vi "DataProcess_CutAndAverage.vi"() -> ()   [LabVIEW 2015]
uses:
  Shared Libraries/CustomVIs/CustomVI.lvlib
  ExpData/ExpData.lvclass
  <vilib>/Utility/miscctls.llb/LVAnnotationListTypeDef.ctl
  EMG/EMG.lvclass
  CAlex2-Data/CAlex2_Data.lvclass
  TypeDef/Control 1.ctl
panel:
  in  "SyncIn":bool
  out "EMGmean":dbl[][](array[numeric])
  in  "Scale(x1)":u16(ring)=15 items=["x1"=1, "x15"=15]
  out "MuscleNum":i32
  in  "FolderOpen":bool
  in  "Tab Control":enum32{"Cut&Average", "Data Process"}(tab)
  in  "EMG Y scale":i32(slide) min=0 max=1000 step=50 scale=0.0..1000.0
  in  "EMGmean-shift":i32(slide) scale=-100.0..100.0
  in  "Reset Display":bool
  in  "Graph-JointAngles":dbl[][](graph)
  out "GaitTraj":cluster{"Mean":dbl[], "Mean":dbl[]}[](graph)
  in  "Graph-EMG":dbl[][](graph)
  in  "SAVE":bool
  in  "Next":bool
  out "EMGmean-display":dbl[][](graph)
  out "AnglesCutted":dbl[][](graph)
  in  "Cur Parameter":dbl=100.0
  in  "Cut Data":bool
  in  "Cut Method":enum16{"Peak", "Valley", "Threshold"}(ring)
  in  "Graph-AnklePos":dbl[][](graph)
  out "Cycle#":dbl format="%#.1f"
  in  "Start Time (s)":dbl=100.0
  in  "End Time (s)":dbl=100.0
  in  "CutVar":enum16{"3D-x", "2D-x"}(ring)
  in  "Open Gait Template":bool
  in  "Gait Template":path
  out "XY Graph":cluster{"X":dbl, "Y":dbl}[](graph)
  in  "EMG":bool
  in  "Save":bool
  out "EMGstd":dbl[][](array[numeric])
  in  "Overwrite":bool
  in  "Search Pattern":string="sub*.txt"
  in  "Output Folder: Averaged & EMG Files":path=path "E:/Dropbox (Lab)/C-ALEX/Experiments"
  in  "Output Folder: Marked Files":path=path "E:/Dropbox (Lab)/C-ALEX/Experiments"
  in  "File List":i32(listbox)
  in  "FolderStop":bool
  in  "EMG":path
  in  "Unmarked Files":path
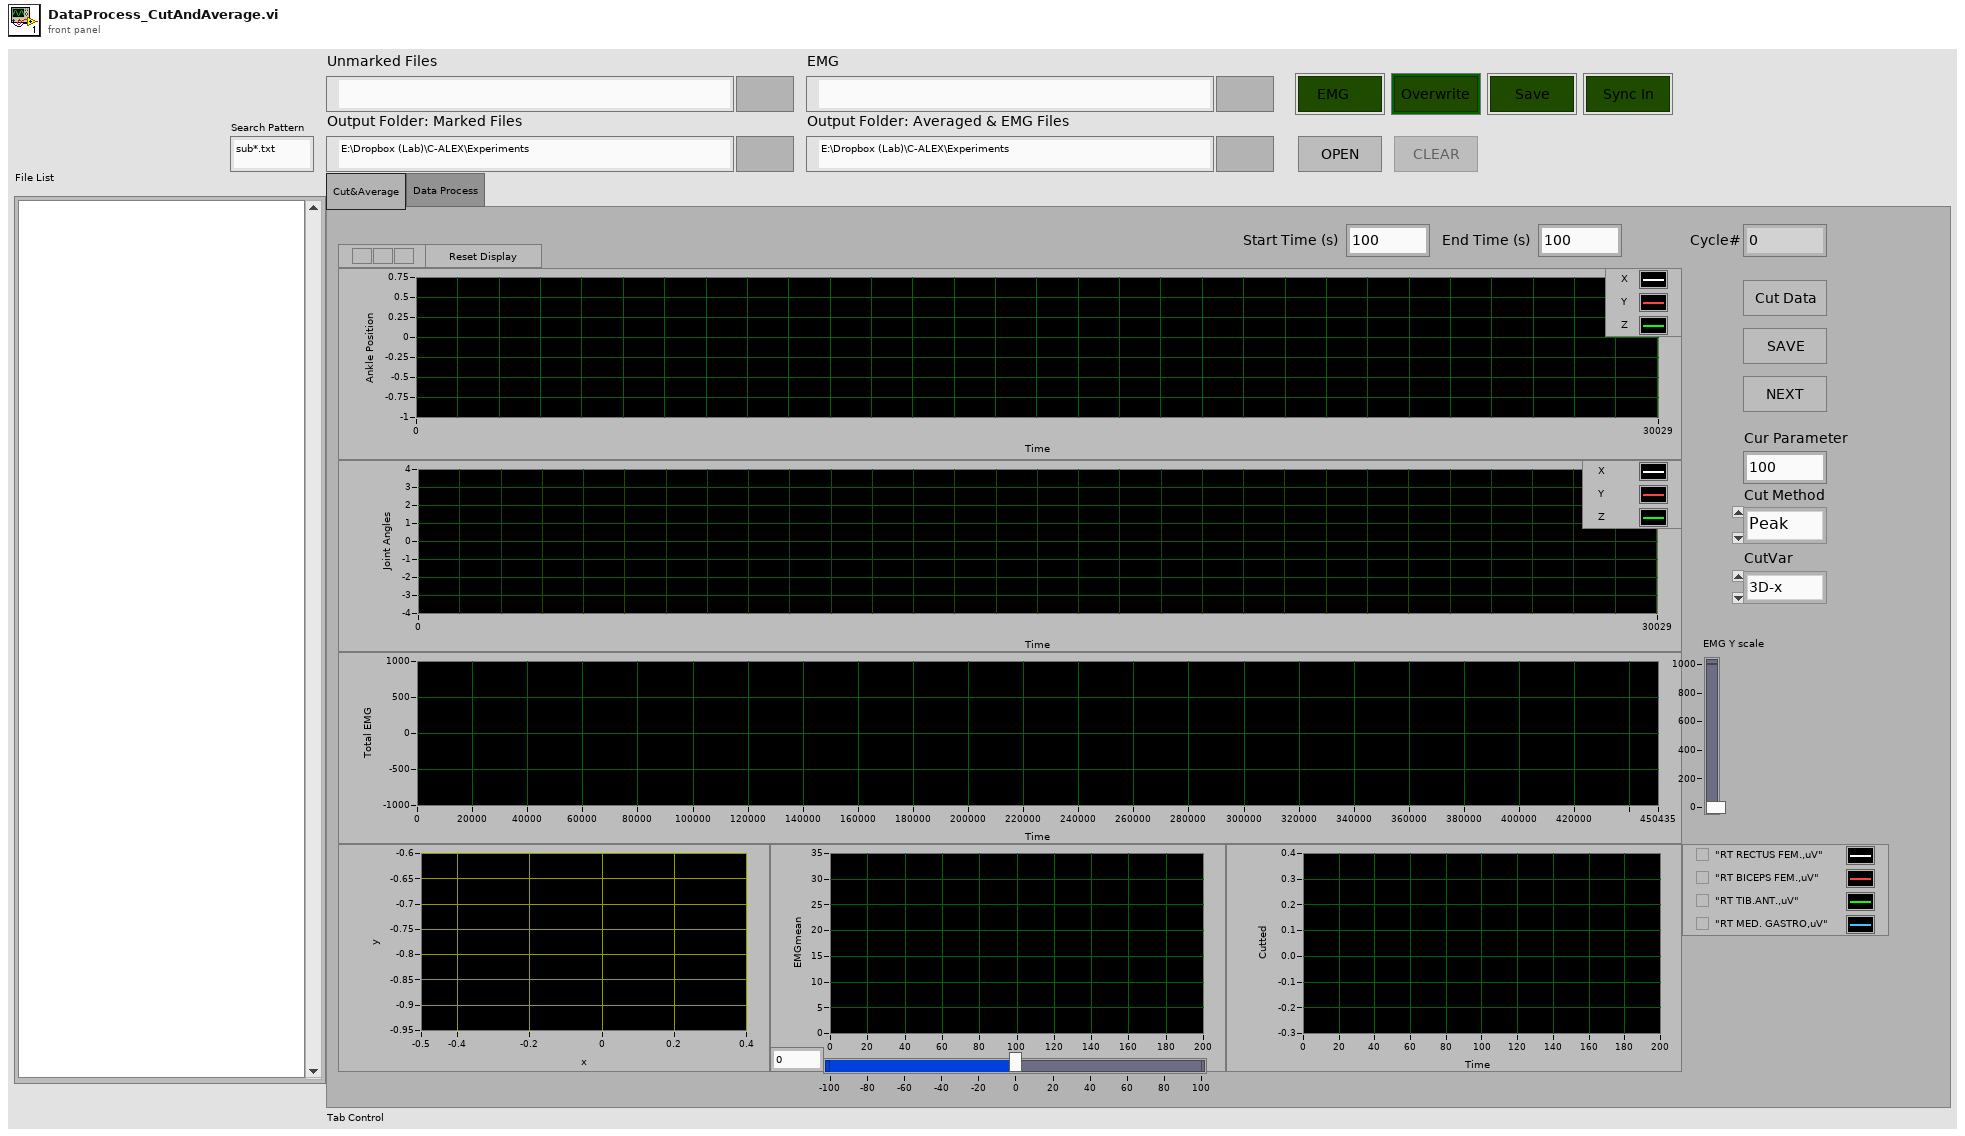
[diagram p1: front panel]
types:
  T1 = typedef "Control 1.ctl" = cluster{"FilePath":path, "ProcParentPath":path, "ResParentPath":path, "EMGPath":path, "CuttedEMGPath":path, "Cutted":bool, "Processed":bool}
  T2 = enum8{"Enabled", "Disabled", "Disabled and Grayed Out"}
  T3 = typedef "LVAnnotationListTypeDef.ctl" = cluster{"Name":string, "Color":u32, "Style":u8, "Point Style":u8, "Name Visible":bool, "Allow Drag":bool, "Annotation Mode":u32, "Plot":i32, "Index":i32, "Position":cluster{"X":dbl, "Y":dbl}, "X Scale":u32, "Y Scale":u32, "Show Arrow":bool, "Lock Name":bool, "Plot Area":i32, "Label Offset":cluster{"X":dbl, "Y":dbl}}[]
  T4 = typedef "LVPoint32TypeDef.ctl" = cluster{"Horizontal":i32, "Vertical":i32}
  T5 = typedef "eventsource.ctl" = u32
  T6 = typedef "LVRangeTypeDef.ctl" = cluster{"Minimum":dbl, "Maximum":dbl, "Increment":dbl, "Minor Increment":dbl, "Start":dbl}
  T7 = cluster{"CuttedData-Concatenated":dbl[], "CuttedData-Concatenated":dbl[]}
  T8 = cluster{"CuttedData-Concatenated":dbl[], "CuttedData-Concatenated":dbl[]}[]
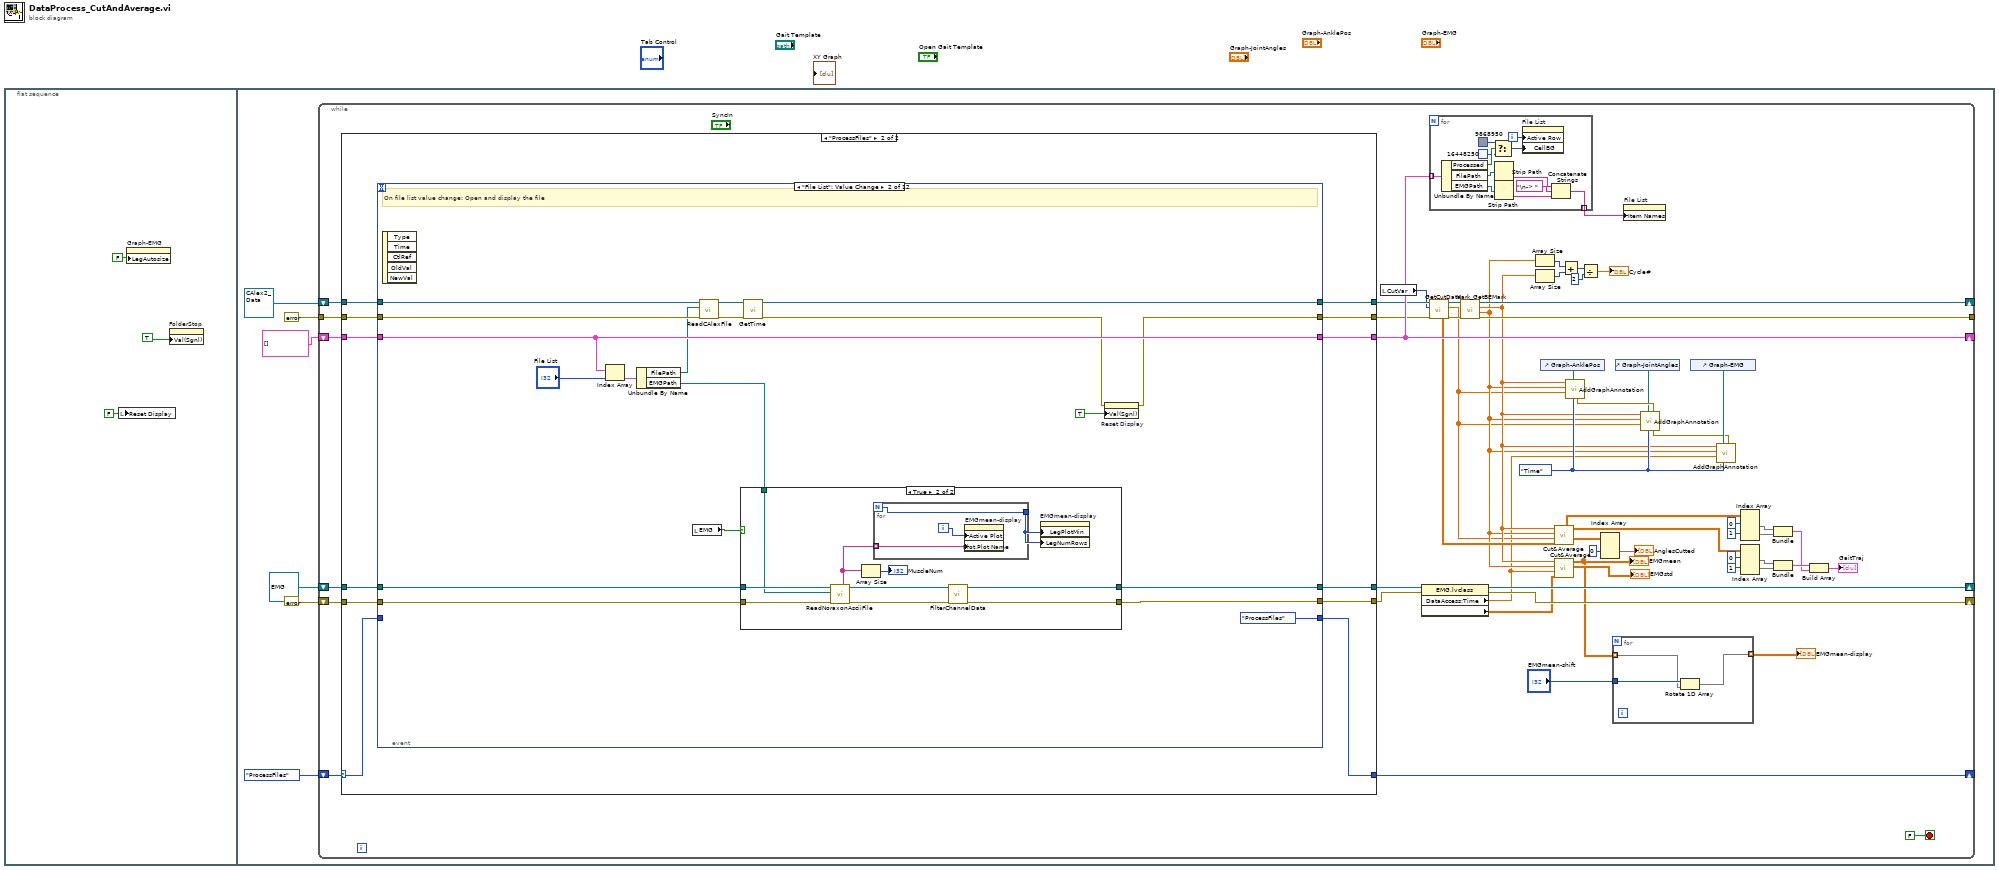
[diagram p0: block diagram]
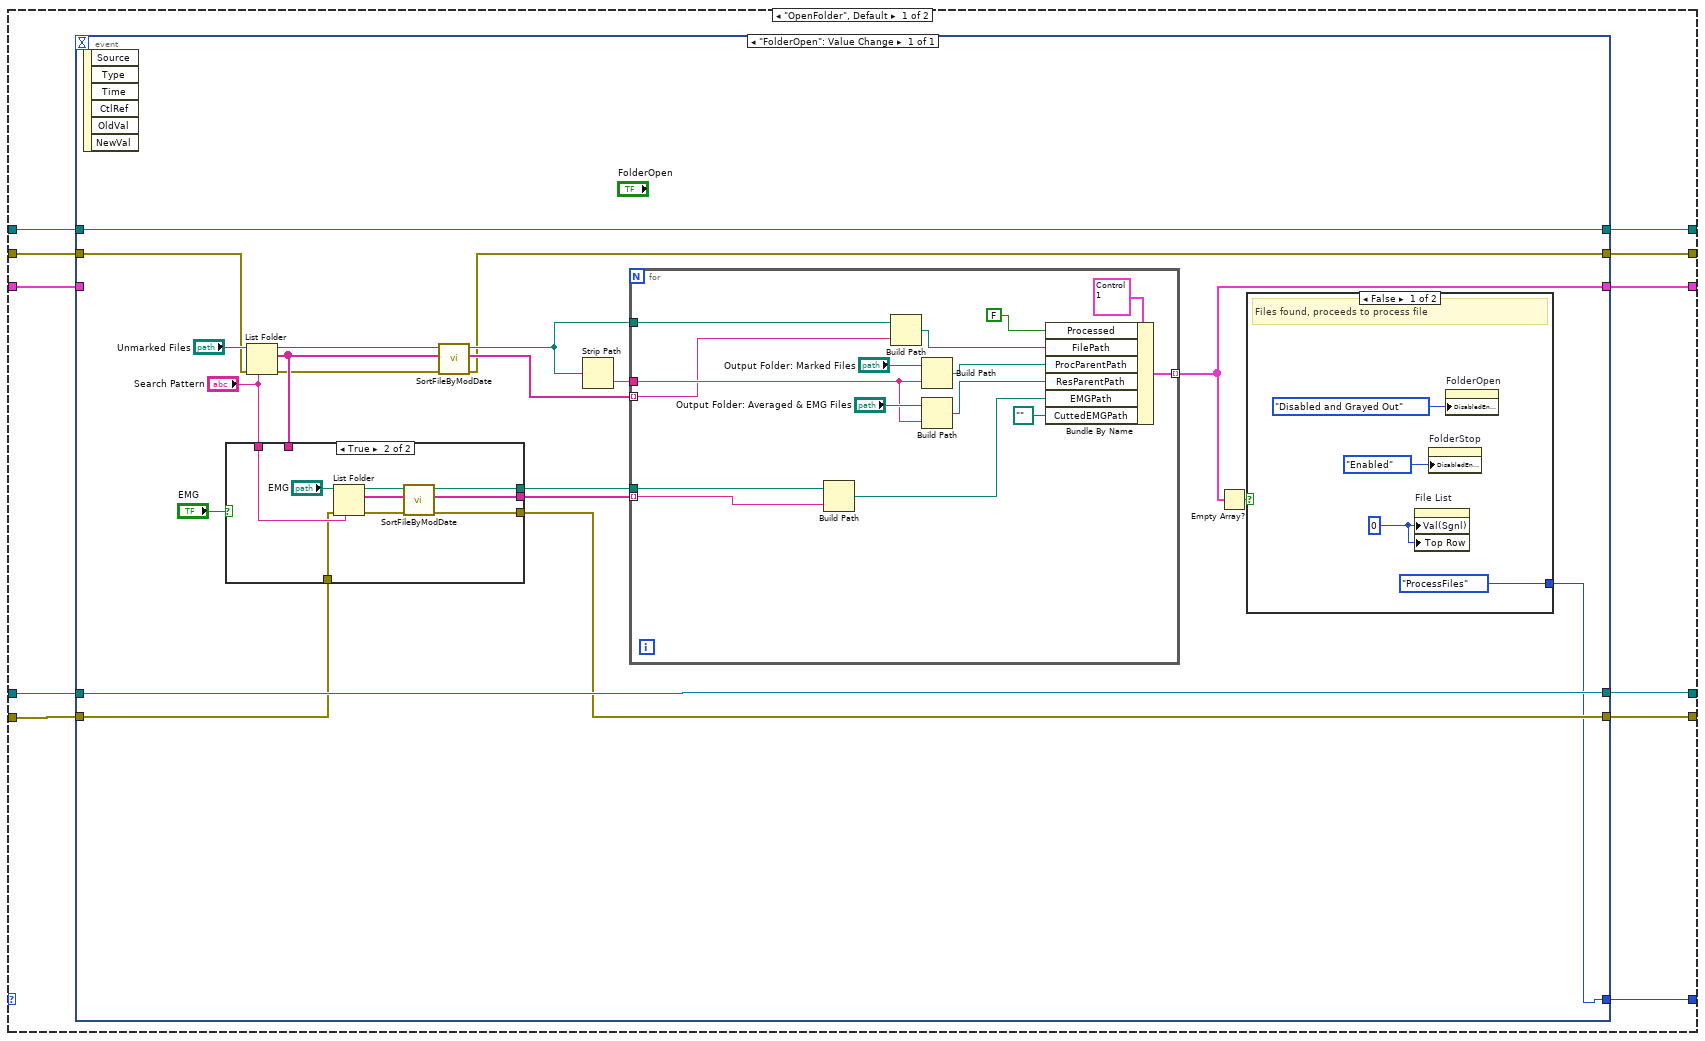
[diagram p2: hidden frame]
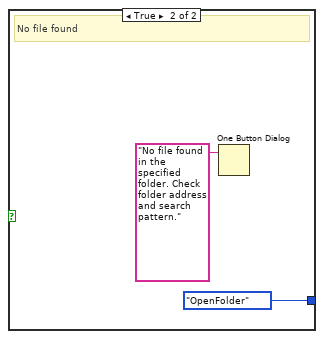
[diagram p3: hidden frame]
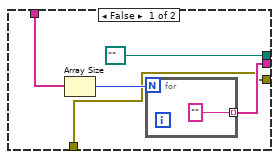
[diagram p4: hidden frame]
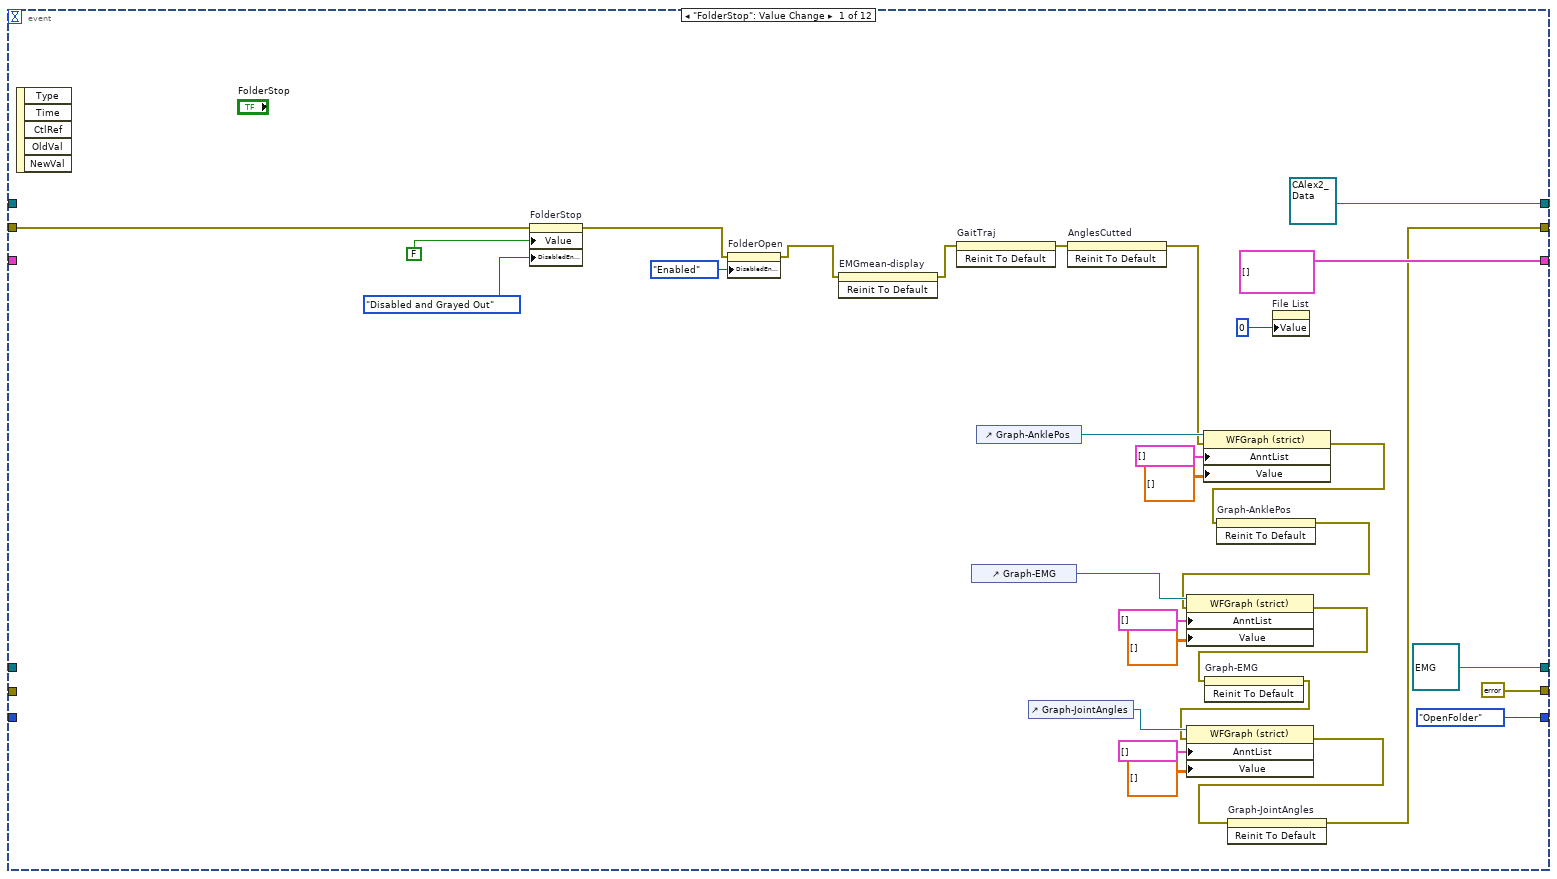
[diagram p5: hidden frame]
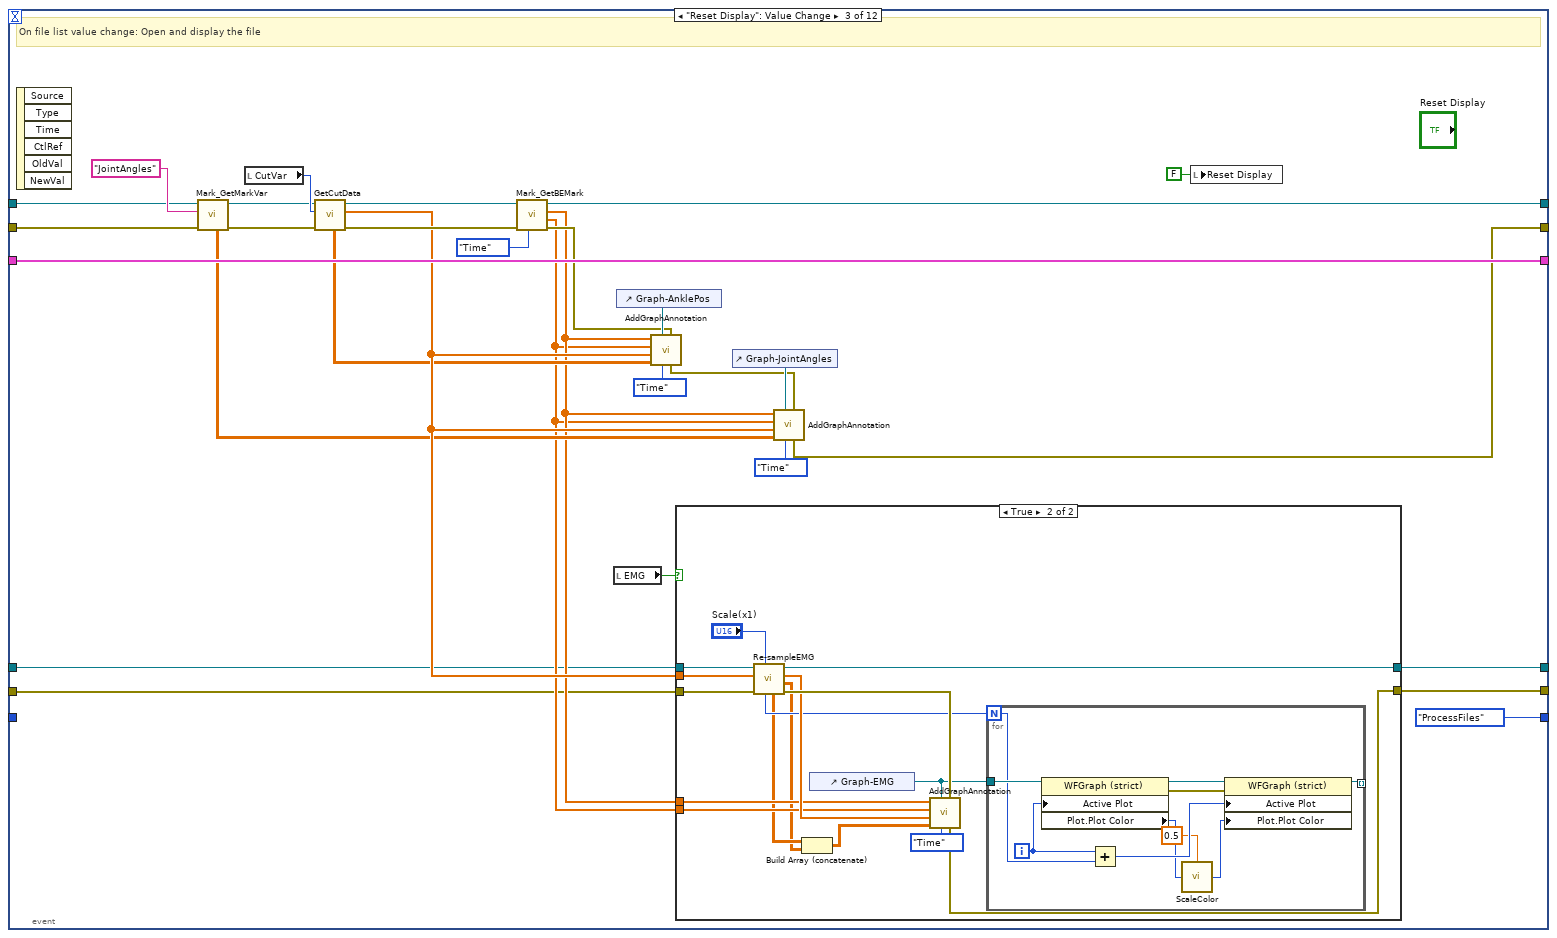
[diagram p7: hidden frame]
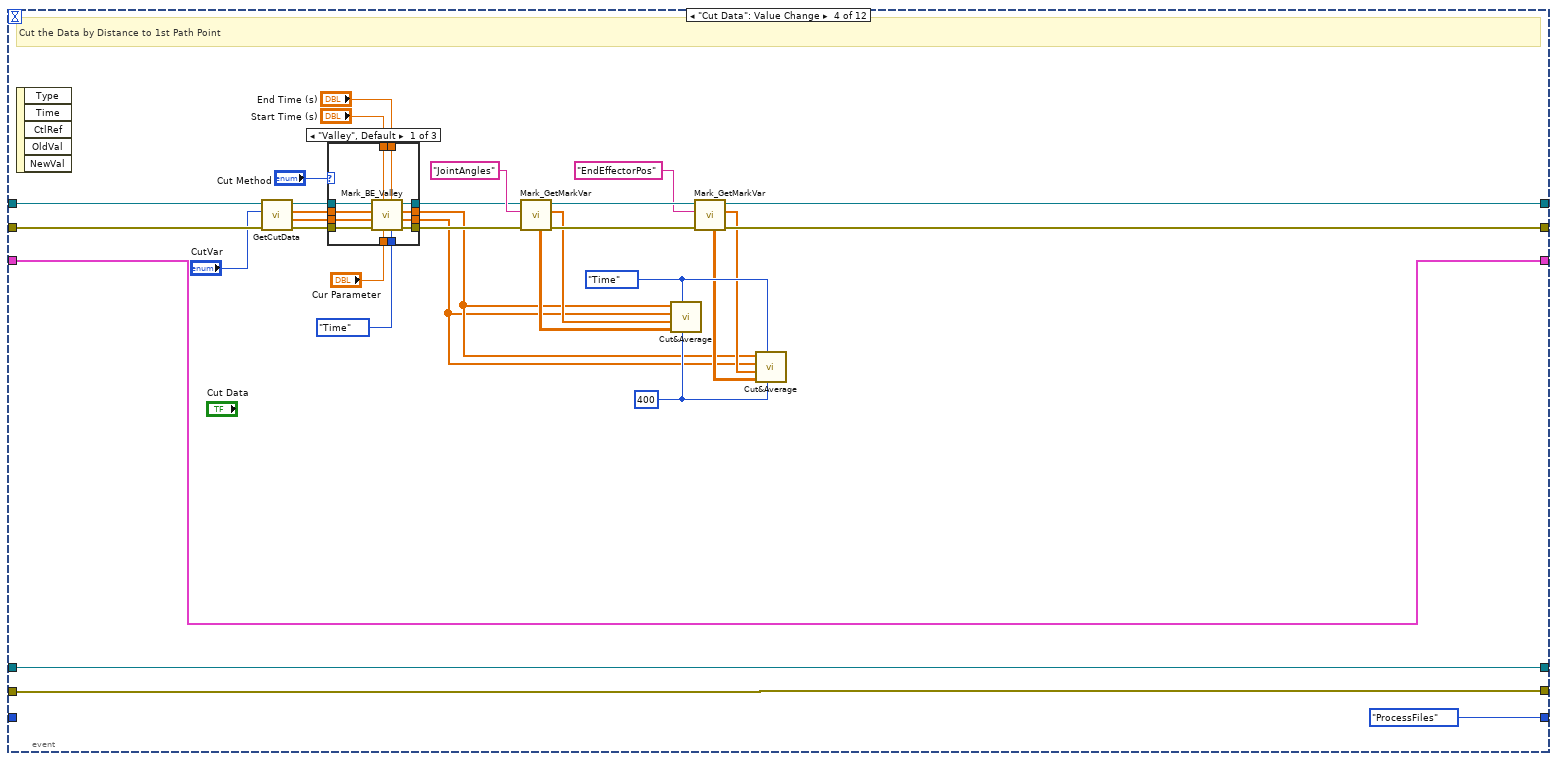
[diagram p9: hidden frame]
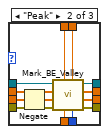
[diagram p10: hidden frame]
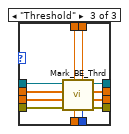
[diagram p11: hidden frame]
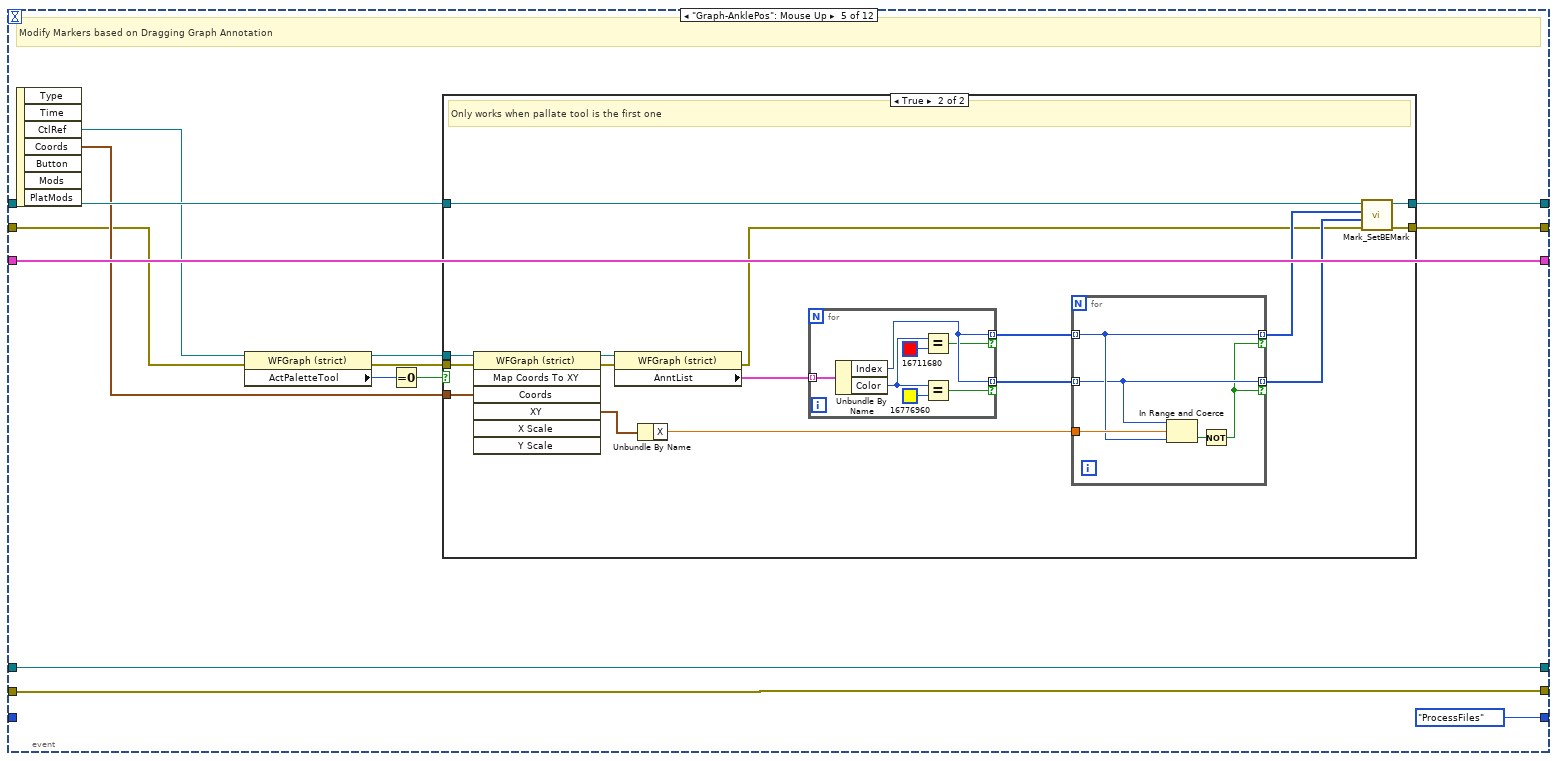
[diagram p12: hidden frame]
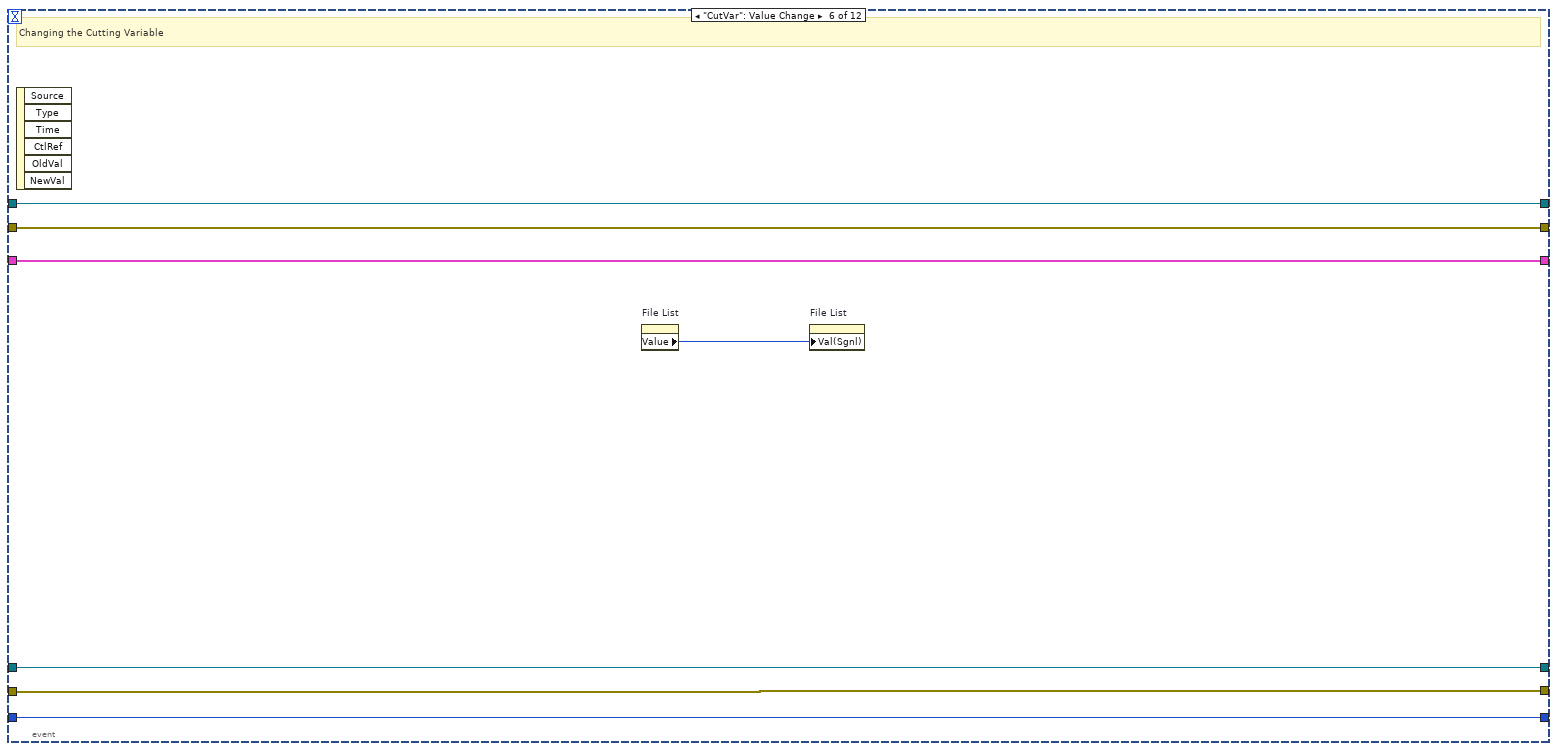
[diagram p14: hidden frame]
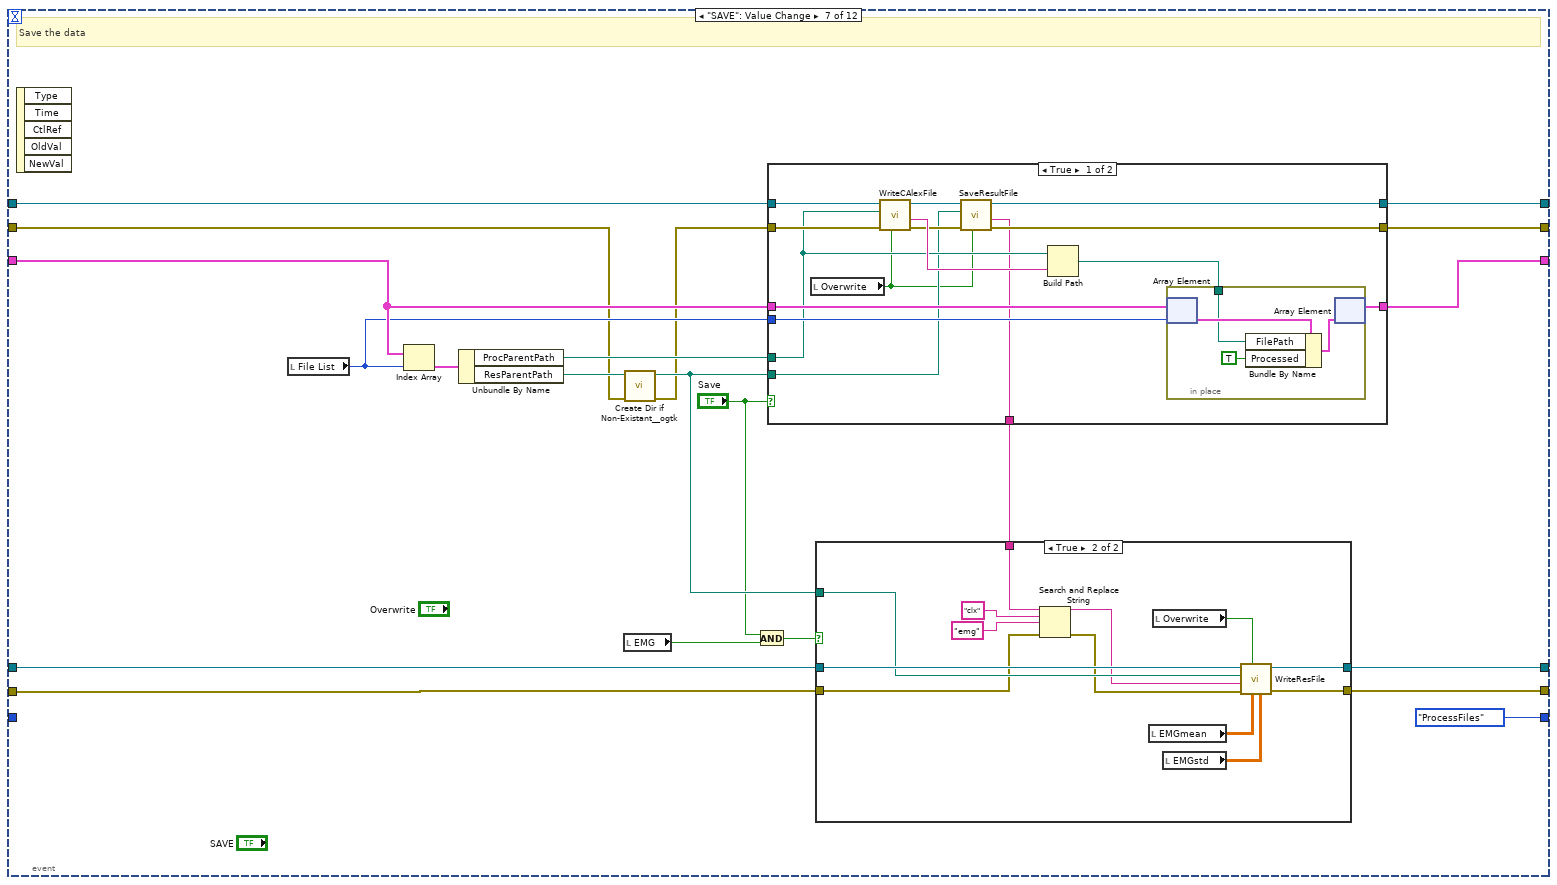
[diagram p15: hidden frame]
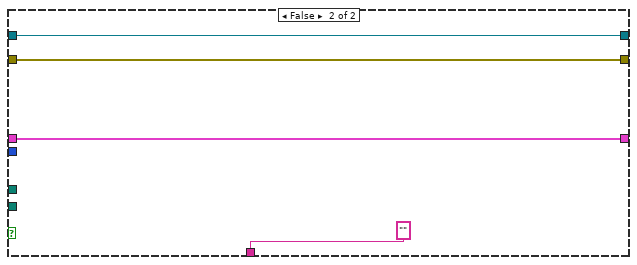
[diagram p17: hidden frame]
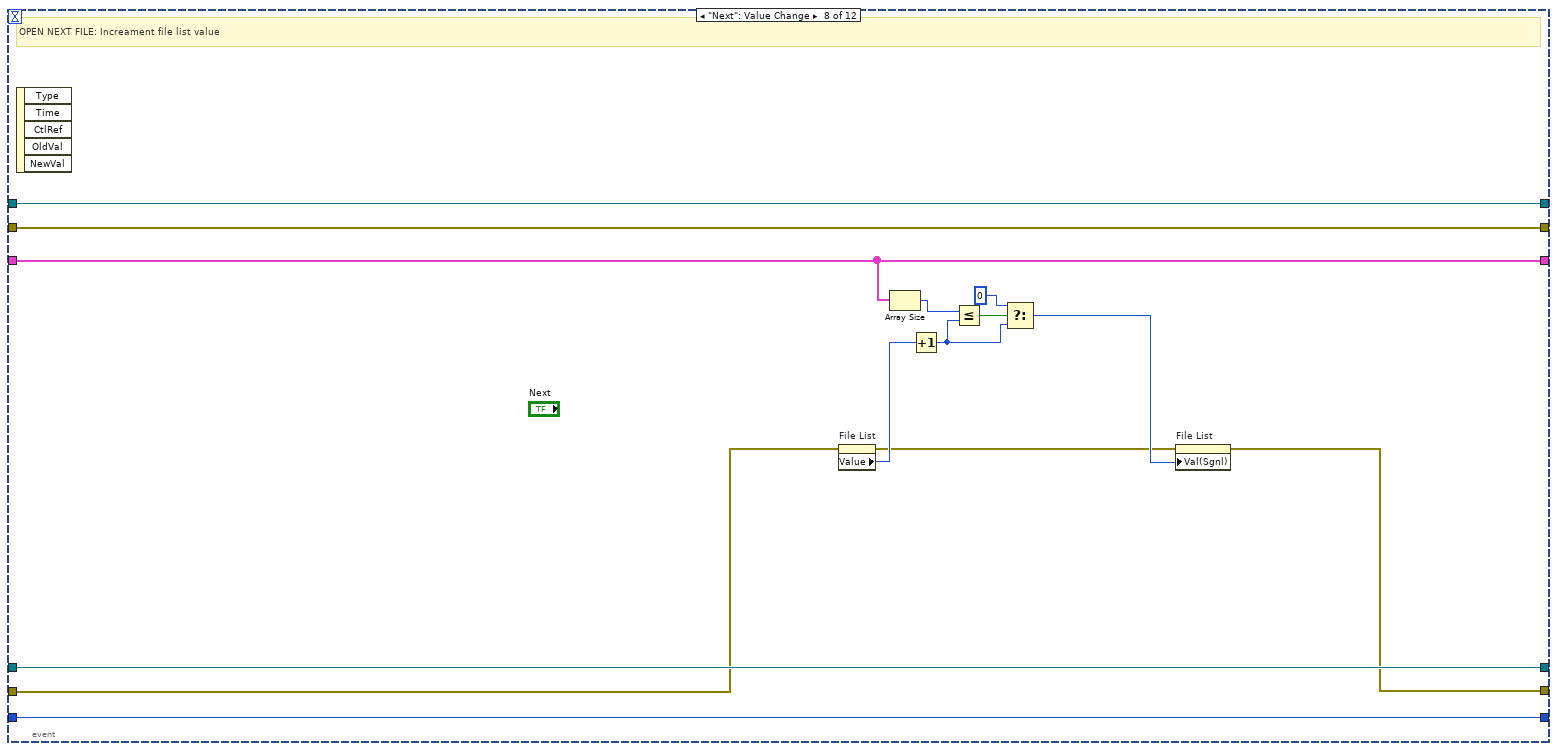
[diagram p18: hidden frame]
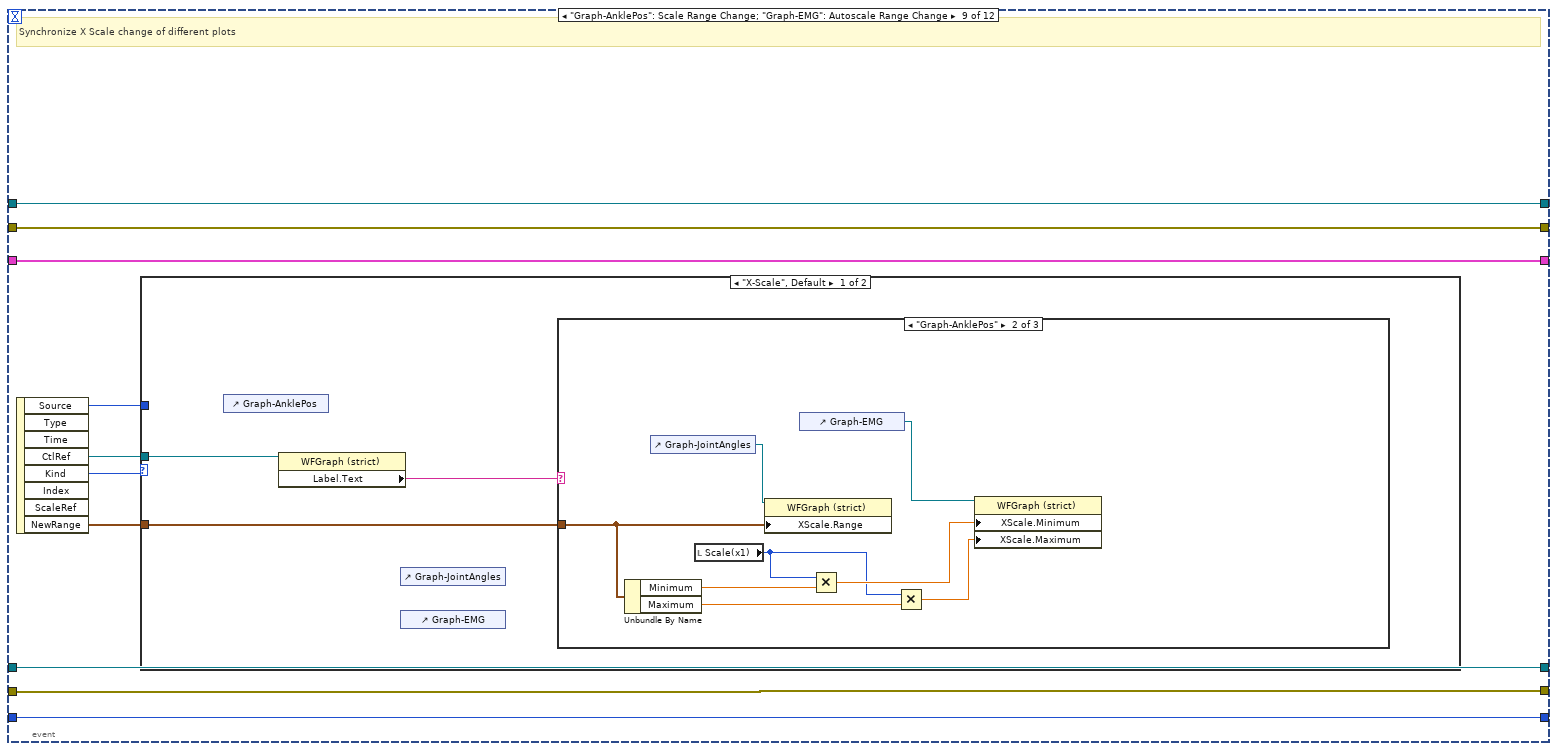
[diagram p19: hidden frame]
diagram:
  n1 = flat-sequence {
    frame #0 {
      n2 = local write "Reset Display"(FALSE ("Reset Display")) -> ()
      n3 = property on="Graph-EMG" class="WFGraph (strict)"("LegAutosize"=FALSE ("Legend:Autosize")) -> ()  [unwired: 2 in, 2 out]
      n4 = property on="FolderStop" class="Bool (strict)"("Val(Sgnl)"=TRUE) -> ()  [unwired: 2 in, 2 out]
    }
    frame #1 {
      n5 = while {
        shift-right: [w61] -> _
        shift-left: enum16{"OpenFolder", "ProcessFiles"}."ProcessFiles" ("State") -> [w39]
        shift-right: [w44] -> _
        shift-left: refnum<class "CAlex2_Data.lvclass"> refnum ("CAlexData") -> [w67]
        shift-right: [w65] -> _
        shift-left: T1[] [] -> [w66]
        tunnel: errorcluster {"status"=FALSE, "code"=0, "source"=""} ("error out") -> [w64]
        tunnel: [w59] -> _
        shift-right: [w54] -> _
        shift-left: refnum<class "EMG.lvclass"> refnum ("EMG.lvclass") -> [w62]
        shift-right: [w52] -> _
        shift-left: errorcluster {"status"=FALSE, "code"=0, "source"=""} ("error out") -> [w60]
        stop <- FALSE stop-if-true
        w18 = enum16{"Time", "Percentage", "Index"}."Time" ("Input Type")
        n6 = case shown="\"ProcessFiles\"" w39 {
          selector: w39 -> [_ w138]
          tunnel: w67 -> [w81 w149]
          tunnel: w66 -> [w79 w148]
          tunnel: [w76 w147] -> w65
          tunnel: w64 -> [w80 w146]
          tunnel: w62 -> [w72 w145]
          tunnel: [w73 w144] -> w61
          tunnel: w60 -> [w71 w143]
          tunnel: [w75 w142] -> w55
          tunnel: [w74 w141] -> w53
          tunnel: [w77 w140] -> w42
          tunnel: [w78 w139] -> w40
          frame "OpenFolder", Default {
            n7 = event shown="[0] \"FolderOpen\": Value Change" {
              selector: _ -> [_]
              dyn-events: _ -> [_]
              timeout: _ -> [_]
              tunnel: w81 -> [w101]
              tunnel: w80 -> [w86]
              tunnel: w79 -> [_]
              tunnel: [w101] -> w78
              tunnel: [w82] -> w77
              tunnel: [w84] -> w76
              tunnel: [w100] -> w75
              tunnel: [w89] -> w74
              tunnel: [w85] -> w73
              tunnel: w72 -> [w100]
              tunnel: w71 -> [w88]
              event "FolderOpen": Value Change {
                n8 = event-data() -> ()  [unwired: 1 in, 6 out]
                n9 = List Folder(path="Unmarked Files", pattern="Search Pattern", error in=w86) -> (path out=w97:path, filenames=w90:string[], error out=w87:errorcluster)  [unwired: 1 in, 1 out]
                n10 = case shown="True" "EMG" {
                  tunnel: [w110 w118] -> w91
                  tunnel: [path "" ("path out") w119] -> w92
                  tunnel: "Search Pattern" -> [_ w121]
                  tunnel: w90 -> [w111 _]
                  tunnel: [w108 w115] -> w89
                  tunnel: w88 -> [w108 w114]
                  frame False {
                    n11 = Array Size(array=w111) -> (size(s)=w109:i32)
                    n12 = for {
                      N: w109 -> [_]
                      tunnel: [""] -> w110 mode=indexing
                    }
                  }
                  frame True {
                    n13 = List Folder(path="EMG", pattern=w121, error in=w114) -> (path out=w120:path, filenames=w117:string[], error out=w116:errorcluster)  [unwired: 1 in, 1 out]
                    n14 = call "SortFileByModDate.vi"("error in (no error)"=w116, "Filenames"=w117, "Parent Path"=w120) -> ("error out"=w115:errorcluster, "Sorted Filenames"=w118:string[], "Parent Path dup"=w119:path)  [unwired: 6 in]
                  }
                }
                n15 = call "SortFileByModDate.vi"("error in (no error)"=w87, "Filenames"=w90, "Parent Path"=w97) -> ("error out"=w82:errorcluster, "Sorted Filenames"=w96:string[], "Parent Path dup"=w95:path)  [unwired: 6 in]
                n16 = Strip Path(path=w95) -> (name=w94:string)  [unwired: 1 out]
                n17 = for {
                  tunnel: w96 -> [w127] mode=indexing
                  tunnel: w91 -> [w123] mode=indexing
                  tunnel: w92 -> [w125]
                  tunnel: w95 -> [w126]
                  tunnel: [w137] -> w84 mode=indexing
                  tunnel: w94 -> [w131]
                  n18 = Build Path(base path=w125, name or relative path=w123) -> (appended path=w124:path)
                  n19 = Build Path(base path=w126, name or relative path=w127) -> (appended path=w128:path)
                  n20 = Build Path(base path="Output Folder: Marked Files", name or relative path=w131) -> (appended path=w134:path)
                  n21 = Build Path(base path="Output Folder: Averaged & EMG Files", name or relative path=w131) -> (appended path=w133:path)
                  n22 = Bundle By Name(cluster=T1 {"FilePath"=path "", "ProcParentPath"=path "", "ResParentPath"=path "", "EMGPath"=path "", "CuttedEMGPath"=path "", "Cutted"=TRUE, "Processed"=FALSE}, "Processed"=FALSE, "FilePath"=w128, "ProcParentPath"=w134, "ResParentPath"=w133, "EMGPath"=w124, "CuttedEMGPath"=path "") -> (w137:T1)
                }
                n23 = Empty Array?(array=w84) -> (empty?=w83:bool)
                n24 = case shown="False" w83 {
                  tunnel: [enum16{"OpenFolder", "ProcessFiles"}."ProcessFiles" ("State") enum16{"OpenFolder", "ProcessFiles"}."OpenFolder" ("State")] -> w85
                  frame False {
                    w105 = 0
                    # "Files found, proceeds to process file"
                    n25 = property on="File List" class="LstBox (strict)"("Val(Sgnl)"=w105, "Top Row"=w105) -> ()  [unwired: 2 in, 2 out]
                    n26 = property on="FolderStop" class="Bool (strict)"("DisabledEnum"=T2."Enabled" ("Disabled")) -> ()  [unwired: 2 in, 2 out]
                    n27 = property on="FolderOpen" class="Bool"("DisabledEnum"=T2."Disabled and Grayed Out" ("Disabled")) -> ()  [unwired: 2 in, 2 out]
                  }
                  frame True {
                    # "No file found"
                    n28 = One Button Dialog(message="No file found in the specified folder. Check folder address and search pattern.") -> ()  [unwired: 1 in, 1 out]
                  }
                }
              }
            }
          }
          frame "ProcessFiles" {
            n29 = event shown="[1] \"File List\": Value Change" {
              selector: _ -> [_ _ _ _ _ _ _ _ _ _ _ _]
              dyn-events: _ -> [_ _ _ _ _ _ _ _ _ _ _ _]
              timeout: _ -> [_ _ _ _ _ _ _ _ _ _ _ _]
              tunnel: [enum16{"OpenFolder", "ProcessFiles"}."OpenFolder" ("State") enum16{"OpenFolder", "ProcessFiles"}."ProcessFiles" ("State") enum16{"OpenFolder", "ProcessFiles"}."ProcessFiles" ("State") enum16{"OpenFolder", "ProcessFiles"}."ProcessFiles" ("State") enum16{"OpenFolder", "ProcessFiles"}."ProcessFiles" ("State") w386 enum16{"OpenFolder", "ProcessFiles"}."ProcessFiles" ("State") w461 w469 w504 w518 w526] -> w144
              tunnel: w149 -> [_ w197 w221 w301 w352 w389 w400 w464 w474 w506 w523 w531]
              tunnel: w148 -> [_ w196 w241 w300 w351 w387 w409 w455 w472 w505 w521 w529]
              tunnel: [T1[] [] w196 w241 w300 w351 w387 w410 w455 w472 w505 w521 w529] -> w147
              tunnel: w138 -> [_ _ _ _ _ w386 _ w461 w469 w504 w518 w526]
              tunnel: [refnum<class "CAlex2_Data.lvclass"> refnum ("CAlexData") w184 w242 w302 w353 w389 w411 w464 w474 w506 w523 w531] -> w139
              tunnel: [w152 w180 w219 w299 w350 w388 w408 w463 w473 w495 w522 w530] -> w140
              tunnel: w146 -> [w161 w195 w220 w298 w344 w388 w394 w463 w473 w496 w522 w530]
              tunnel: w145 -> [_ w194 w215 w297 w349 w390 w406 w462 w471 w501 w520 w528]
              tunnel: w143 -> [_ w193 w214 w296 w348 w391 w404 w452 w470 w499 w519 w527]
              tunnel: [refnum<class "EMG.lvclass"> refnum ("EMG.lvclass") w192 w240 w297 w349 w390 w407 w462 w471 w500 w520 w528] -> w142
              tunnel: [errorcluster {"status"=FALSE, "code"=0, "source"=""} ("error in (no error)") w191 w239 w296 w348 w391 w405 w451 w470 w498 w519 w527] -> w141
              event "FolderStop": Value Change {
                n30 = event-data() -> ()  [unwired: 1 in, 5 out]
                n31 = property on="FolderStop" class="Bool (strict)"(error in=w161, "Value"=FALSE, "DisabledEnum"=T2."Disabled and Grayed Out" ("Disabled")) -> (error out=w160:errorcluster)  [unwired: 1 in, 1 out]
                n32 = property on="FolderOpen" class="Bool"(error in=w160, "DisabledEnum"=T2."Enabled" ("Disabled")) -> (error out=w151:errorcluster)  [unwired: 1 in, 1 out]
                n33 = invoke on="EMGmean-display" class="WFGraph (strict)" method="Reinit To Default"(error in=w151) -> (error out=w150:errorcluster)  [unwired: 2 in, 2 out]
                n34 = invoke on="GaitTraj" class="XYGraph (strict)" method="Reinit To Default"(error in=w150) -> (error out=w163:errorcluster)  [unwired: 2 in, 2 out]
                n35 = control-ref of="Graph-EMG"() -> (w170:refnum<vi>)
                n36 = control-ref of="Graph-AnklePos"() -> (w175:refnum<vi>)
                n37 = control-ref of="Graph-JointAngles"() -> (w164:refnum<vi>)
                n38 = invoke on="AnglesCutted" class="WFGraph (strict)" method="Reinit To Default"(error in=w163) -> (error out=w162:errorcluster)  [unwired: 2 in, 2 out]
                n39 = property class="WFGraph (strict)"(reference=w175, error in=w162, "AnntList"=T3 [] ("Annotation List"), "Value"=dbl[][] []) -> (error out=w157:errorcluster)  [unwired: 1 out]
                n40 = invoke on="Graph-AnklePos" class="WFGraph (strict)" method="Reinit To Default"(error in=w157) -> (error out=w156:errorcluster)  [unwired: 2 in, 2 out]
                n41 = property class="WFGraph (strict)"(reference=w170, error in=w156, "AnntList"=T3 [] ("Annotation List"), "Value"=dbl[][] []) -> (error out=w155:errorcluster)  [unwired: 1 out]
                n42 = invoke on="Graph-EMG" class="WFGraph (strict)" method="Reinit To Default"(error in=w155) -> (error out=w154:errorcluster)  [unwired: 2 in, 2 out]
                n43 = property class="WFGraph (strict)"(reference=w164, error in=w154, "AnntList"=T3 [] ("Annotation List"), "Value"=dbl[][] []) -> (error out=w153:errorcluster)  [unwired: 1 out]
                n44 = invoke on="Graph-JointAngles" class="WFGraph (strict)" method="Reinit To Default"(error in=w153) -> (error out=w152:errorcluster)  [unwired: 2 in, 2 out]
                n45 = property on="File List" class="LstBox (strict)"("Value"=0) -> ()  [unwired: 2 in, 2 out]
              }
              event "File List": Value Change {
                # "On file list value change: Open and display the file"
                n46 = event-data() -> ()  [unwired: 1 in, 5 out]
                n47 = Index Array(array=w196, index="File List") -> (element=w190:T1)
                n48 = Unbundle By Name(w190) -> ("FilePath"=w189:path, "EMGPath"=w187:path)
                n49 = local read "EMG"() -> (w186:bool)
                n50 = call "ReadCAlexFile.vi"("error in (no error)"=w195, "ExpData File Path"=w189, "CAlexData2"=w197) -> ("error out"=w183:errorcluster, "CAlexData 2"=w185:refnum<class "CAlex2_Data.lvclass">)  [unwired: 7 in]
                n51 = case shown="True" w186 {
                  tunnel: w194 -> [w200 w210]
                  tunnel: w193 -> [w199 w209]
                  tunnel: [w200 w204] -> w192
                  tunnel: [w199 w202] -> w191
                  tunnel: w187 -> [_ w208]
                  frame False {
                  }
                  frame True {
                    n52 = call "ReadNoraxonAsciiFile.vi"("error in (no error)"=w209, "Path"=w208, "EMG in"=w210) -> ("error out"=w203:errorcluster, "EMG out"=w205:refnum<class "EMG.lvclass">, "Muscle Names"=w207:string[])  [unwired: 4 in, 2 out]
                    n53 = Array Size(array=w207) -> (size(s)=→"MuscleNum":i32)
                    n54 = for {
                      N -> [w211]
                      tunnel: w207 -> [w213] mode=indexing
                      tunnel: [w211] -> w201
                      i -> [w212]
                      n55 = property on="EMGmean-display" class="WFGraph (strict)"("Active Plot"=w212, "Plot.Plot Name"=w213) -> ()  [unwired: 2 in, 2 out]
                    }
                    n56 = call "FilterChannelData.vi"("error in (no error)"=w203, "EMG in"=w205) -> ("error out"=w202:errorcluster, "EMG out"=w204:refnum<class "EMG.lvclass">)  [unwired: 7 in, 1 out]
                    n57 = property on="EMGmean-display" class="WFGraph (strict)"("LegPlotMin"=w201, "LegNumRows"=w201) -> ()  [unwired: 2 in, 2 out]
                  }
                }
                n58 = call "GetTime.vi"("error in (no error)"=w183, "CarexMData in"=w185) -> ("error out"=w181:errorcluster, "CarexMData out"=w184:refnum<class "CAlex2_Data.lvclass">)  [unwired: 7 in, 1 out]
                n59 = property on="Reset Display" class="Bool (strict)"(error in=w181, "Val(Sgnl)"=TRUE) -> (error out=w180:errorcluster)  [unwired: 1 in, 1 out]
              }
              event "Reset Display": Value Change {
                # "On file list value change: Open and display the file"
                n60 = event-data() -> ()  [unwired: 1 in, 6 out]
                n61 = call "Mark_GetMarkVar.vi"("error in (no error)"=w220, "VarName"="JointAngles" ("Name"), "ExpData in"=w221) -> ("error out"=w227:errorcluster, "ExpData out"=w228:refnum<class "CAlex2_Data.lvclass">, "Var_All"=w226:dbl[][])  [unwired: 4 in, 2 out]
                n62 = local read "CutVar"() -> (w232:enum16{"3D-x", "2D-x"})
                n63 = call "GetCutData.vi"("error in (no error)"=w227, "CutVar"=w232, "CAlexData"=w228) -> ("error out"=w237:errorcluster, "Time"=w231:dbl[], "CAlexData out"=w238:refnum<class "CAlex2_Data.lvclass">, "MarkingVar3"=w229:dbl[][])  [unwired: 4 in, 1 out]
                n64 = call "Mark_GetBEMark.vi"("Type (Time)"=enum16{"Time", "Percentage", "Index"}."Time" ("Output Type (Time)"), "error in (no error)"=w237, "ExpData In"=w238) -> ("error out"=w222:errorcluster, "End"=w217:dbl[], "Begin"=w218:dbl[], "ExpData Out"=w242:refnum<class "CAlex2_Data.lvclass">)  [unwired: 4 in, 1 out]
                n65 = local read "EMG"() -> (w233:bool)
                n66 = control-ref of="Graph-AnklePos"() -> (w236:refnum<vi>)
                n67 = call "AddGraphAnnotation.vi"("error in (no error)"=w222, "Input Type (Time)"=enum16{"Time", "Percentage", "Index"}."Time" ("Input Type"), "WaveformGraph in"=w236, "Array"=w229, "Time"=w231, "Valleys  (Yellow)"=w217, "Peaks (Red)"=w218) -> ("error out"=w223:errorcluster)  [unwired: 3 in, 1 out]
                n68 = case shown="True" w233 {
                  tunnel: w215 -> [w245 w261]
                  tunnel: w214 -> [w244 w259]
                  tunnel: [w245 w260] -> w240
                  tunnel: [w244 w255] -> w239
                  tunnel: w231 -> [_ w258]
                  tunnel: w218 -> [_ w253]
                  tunnel: w217 -> [_ w252]
                  frame False {
                  }
                  frame True {
                    n69 = call "Re-sampleEMG.vi"("Down Sample External Time (x1)"="Scale(x1)", "error in (no error)"=w259, "External Time"=w258, "EMG in"=w261) -> ("error out"=w256:errorcluster, "EMG"=w246:dbl[][], "Re Sample Time"=w254:dbl[], "EMG out"=w260:refnum<class "EMG.lvclass">, "EMGProcessed"=w247:dbl[][], "ChannelNumber"=w249:i32)  [unwired: 2 in]
                    n70 = Build Array (concatenate)(w247, w246) -> (w250:dbl[][])
                    n71 = control-ref of="Graph-EMG"() -> (w251:refnum<vi>)
                    n72 = call "AddGraphAnnotation.vi"("error in (no error)"=w256, "Input Type (Time)"=enum16{"Time", "Percentage", "Index"}."Time" ("Input Type"), "WaveformGraph in"=w251, "Array"=w250, "Time"=w254, "Valleys  (Yellow)"=w252, "Peaks (Red)"=w253) -> ("error out"=w255:errorcluster)  [unwired: 3 in, 1 out]
                    n73 = for {
                      N: w249 -> [w268]
                      tunnel: w251 -> [w271]
                      tunnel: [w266] -> _ mode=indexing
                      i -> [w265]
                      n74 = property class="WFGraph (strict)"(reference=w271, "Active Plot"=w265) -> (reference out=w270:refnum<vi>, error out=w267:errorcluster, "Plot.Plot Color"=w264:u32)  [unwired: 1 in]
                      n75 = Add(x=w265, y=w268) -> (x+y=w269:i32)
                      n76 = call "ScaleColor.vi"("Scale"=0.5, "Color Box"=w264) -> ("Color Box 2"=w263:u32)  [unwired: 2 in]
                      n77 = property class="WFGraph (strict)"(reference=w270, error in=w267, "Active Plot"=w269, "Plot.Plot Color"=w263) -> (reference out=w266:refnum<vi>)  [unwired: 1 out]
                    }
                  }
                }
                n78 = control-ref of="Graph-JointAngles"() -> (w224:refnum<vi>)
                n79 = call "AddGraphAnnotation.vi"("error in (no error)"=w223, "Input Type (Time)"=enum16{"Time", "Percentage", "Index"}."Time", "WaveformGraph in"=w224, "Array"=w226, "Time"=w231, "Valleys  (Yellow)"=w217, "Peaks (Red)"=w218) -> ("error out"=w219:errorcluster)  [unwired: 3 in, 1 out]
                n80 = local write "Reset Display"(FALSE ("Reset Display")) -> ()
              }
              event "Cut Data": Value Change {
                w286 = 400 ("Dilate Length")
                w287 = enum16{"Time", "Percentage", "Index"}."Time" ("Input Type (Time)")
                # "Cut the Data by Distance to 1st Path Point"
                n81 = event-data() -> ()  [unwired: 1 in, 5 out]
                n82 = call "GetCutData.vi"("error in (no error)"=w298, "CutVar"="CutVar", "CAlexData"=w301) -> ("error out"=w294:errorcluster, "MarkingVar"=w279:dbl[], "Time"=w272:dbl[], "CAlexData out"=w295:refnum<class "CAlex2_Data.lvclass">)  [unwired: 4 in, 1 out]
                n83 = case shown="\"Valley\", Default" "Cut Method" {
                  tunnel: [w315 w328 w337] -> w280
                  tunnel: [w314 w327 w340] -> w281
                  tunnel: w295 -> [w313 w326 w335]
                  tunnel: w294 -> [w312 w325 w332]
                  tunnel: [w311 w324 w339] -> w274
                  tunnel: [w310 w323 w338] -> w273
                  tunnel: "Cur Parameter" -> [w307 w321 w336]
                  tunnel: w272 -> [w309 w317 w334]
                  tunnel: w279 -> [w308 w322 w333]
                  tunnel: enum16{"Time", "Percentage", "Index"}."Time" ("Output Type") -> [w306 w320 w331]
                  tunnel: "Start Time (s)" -> [w305 w319 w330]
                  tunnel: "End Time (s)" -> [w304 w318 w329]
                  frame "Valley", Default {
                    n84 = call "Mark_BE_Valley.vi"("Output Type"=w306, "End Time"=w304, "HalfWidth"=w307, "Start Time"=w305, "error in (no error)"=w312, "Input"=w308, "Time"=w309, "CarexData In"=w313) -> ("error out"=w315:errorcluster, "End"=w310:dbl[], "Begin"=w311:dbl[], "CarexData Out"=w314:refnum<class "CAlex2_Data.lvclass">)
                  }
                  frame "Peak" {
                    n85 = Negate(x=w322) -> (-x=w316:dbl[])
                    n86 = call "Mark_BE_Valley.vi"("Output Type"=w320, "End Time"=w318, "HalfWidth"=w321, "Start Time"=w319, "error in (no error)"=w325, "Input"=w316, "Time"=w317, "CarexData In"=w326) -> ("error out"=w328:errorcluster, "End"=w323:dbl[], "Begin"=w324:dbl[], "CarexData Out"=w327:refnum<class "CAlex2_Data.lvclass">)
                  }
                  frame "Threshold" {
                    n87 = call "Mark_BE_Thrd.vi"("Output Type"=w331, "End Time"=w329, "threshold"=w336, "Start Time"=w330, "error in (no error)"=w332, "Input"=w333, "Time"=w334, "CarexData In"=w335) -> ("error out"=w337:errorcluster, "End"=w338:dbl[], "Begin"=w339:dbl[], "CarexData Out"=w340:refnum<class "CAlex2_Data.lvclass">)
                  }
                }
                n88 = call "Mark_GetMarkVar.vi"("error in (no error)"=w280, "VarName"="JointAngles" ("MarkingVar"), "ExpData in"=w281) -> ("error out"=w290:errorcluster, "Time"=w285:dbl[], "ExpData out"=w291:refnum<class "CAlex2_Data.lvclass">, "Var_All"=w284:dbl[][])  [unwired: 4 in, 1 out]
                n89 = call "Cut&Average.vi"("Dilate Length (200)"=w286, "Input Type (Time)"=w287, "Data"=w284, "Time"=w285, "End"=w273, "Begin"=w274) -> ()  [unwired: 6 out]
                n90 = call "Mark_GetMarkVar.vi"("error in (no error)"=w290, "VarName"="EndEffectorPos" ("MarkingVar"), "ExpData in"=w291) -> ("error out"=w299:errorcluster, "Time"=w283:dbl[], "ExpData out"=w302:refnum<class "CAlex2_Data.lvclass">, "Var_All"=w282:dbl[][])  [unwired: 4 in, 1 out]
                n91 = call "Cut&Average.vi"("Dilate Length (200)"=w286, "Input Type (Time)"=w287, "Data"=w282, "Time"=w283, "End"=w273, "Begin"=w274) -> ()  [unwired: 6 out]
              }
              event "Graph-AnklePos": Mouse Up {
                # "Modify Markers based on Dragging Graph Annotation"
                n92 = event-data() -> ("CtlRef"=w346:refnum<vi>, "Coords"=w347:T4)  [unwired: 1 in, 5 out]
                n93 = property class="WFGraph (strict)"(reference=w346, error in=w344) -> (reference out=w345:refnum<vi>, error out=w343:errorcluster, "ActPaletteTool"=w341:i32)
                n94 = Equal To 0?(x=w341) -> (x = 0?=w342:bool)
                n95 = case shown="True" w342 {
                  tunnel: [w356 w372] -> w353
                  tunnel: w352 -> [w356 w371]
                  tunnel: [w355 w370] -> w350
                  tunnel: w347 -> [_ w368]
                  tunnel: w345 -> [_ w358]
                  tunnel: w343 -> [w355 w357]
                  frame False {
                  }
                  frame True {
                    # "Only works when pallate tool is the first one"
                    n96 = invoke class="WFGraph (strict)" method="Map Coords To XY"(reference=w358, error in=w357, "Coords"=w368) -> (reference out=w366:refnum<vi>, error out=w365:errorcluster, "XY"=w367:cluster{"X":dbl, "Y":dbl})  [unwired: 4 in, 4 out]
                    n97 = property class="WFGraph (strict)"(reference=w366, error in=w365) -> (error out=w359:errorcluster, "AnntList"=w369:T3)  [unwired: 1 out]
                    n98 = Unbundle By Name(w367) -> ("X"=w362:dbl)
                    n99 = for {
                      tunnel: w369 -> [w384] mode=indexing
                      tunnel: [w383] -> w364 mode=indexing if=w380
                      tunnel: [w383] -> w363 mode=indexing if=w378
                      n100 = Unbundle By Name(w384) -> ("Index"=w383:i32, "Color"=w379:u32)
                      n101 = Equal?(x=w379, y=u32 16711680) -> (x = y?=w380:bool)
                      n102 = Equal?(x=w379, y=u32 16776960) -> (x = y?=w378:bool)
                    }
                    n103 = for {
                      tunnel: w364 -> [w376] mode=indexing
                      tunnel: w363 -> [w375] mode=indexing
                      tunnel: w362 -> [w377]
                      tunnel: [w376] -> w361 mode=indexing if=w374
                      tunnel: [w375] -> w360 mode=indexing if=w374
                      n104 = In Range and Coerce(upper limit=w375, x=w377, lower limit=w376) -> (In Range?=w373:bool)  [unwired: 1 out]
                      n105 = Not(x=w373) -> (.not. x?=w374:bool)
                    }
                    n106 = call "Mark_SetBEMark.vi"("error in (no error)"=w359, "End"=w360, "Begin"=w361, "CarexData In"=w371) -> ("error out"=w370:errorcluster, "CarexData Out"=w372:refnum<class "CAlex2_Data.lvclass">)  [unwired: 6 in]
                  }
                }
              }
              event "CutVar": Value Change {
                # "Changing the Cutting Variable"
                n107 = event-data() -> ()  [unwired: 1 in, 6 out]
                n108 = property on="File List" class="LstBox (strict)"() -> ("Value"=w385:i32)  [unwired: 2 in, 2 out]
                n109 = property on="File List" class="LstBox (strict)"("Val(Sgnl)"=w385) -> ()  [unwired: 2 in, 2 out]
              }
              event "SAVE": Value Change {
                # "Save the data"
                n110 = event-data() -> ()  [unwired: 1 in, 5 out]
                n111 = local read "File List"() -> (w401:i32)
                n112 = Index Array(array=w409, index=w401) -> (element=w403:T1)
                n113 = Unbundle By Name(w403) -> ("ProcParentPath"=w402:path, "ResParentPath"=w399:path)
                n114 = local read "EMG"() -> (w395:bool)
                n115 = call <userlib>:"Create Dir if Non-Existant__ogtk.vi"("error in (no error)"=w394, "Directory Path"=w399) -> ("error out"=w393:errorcluster, "dup Directory Path"=w398:path)  [unwired: 7 in, 1 out]
                n116 = And(x="Save", y=w395) -> (x .and. y?=w397:bool)
                n117 = case shown="True" "Save" {
                  tunnel: w400 -> [w436 w450]
                  tunnel: w393 -> [w442 w449]
                  tunnel: [w433 w450] -> w411
                  tunnel: [w432 w449] -> w408
                  tunnel: [w441 w448] -> w410
                  tunnel: w409 -> [w440 w448]
                  tunnel: w402 -> [w431 _]
                  tunnel: w401 -> [w438 _]
                  tunnel: w398 -> [w430 _]
                  tunnel: [w428 "" ("FileName")] -> w392
                  frame True {
                    n118 = local read "Overwrite"() -> (w429:bool)
                    n119 = call "WriteCAlexFile.vi"("Overwrite?(F)"=w429, "error in (no error)"=w442, "Output Path"=w431, "CAlexData"=w436) -> ("error out"=w434:errorcluster, "Actual File Name"=w437:string, "CAlexData 2"=w435:refnum<class "CAlex2_Data.lvclass">)  [unwired: 4 in, 1 out]
                    n120 = call-dynamic "SaveResultFile.vi"("Overwrite"=w429, "error in (no error)"=w434, "FolderPath"=w430, "CAlexData2 in"=w435) -> ("error out"=w432:errorcluster, "FileName"=w428:string, "CAlexData2 out"=w433:refnum<class "CAlex2_Data.lvclass">)  [unwired: 4 in, 1 out]
                    n121 = Build Path(base path=w431, name or relative path=w437) -> (appended path=w439:path)
                    n122 = in-place {
                      in-place-border: w439 -> [w444]
                      n123 = in-place-array #1(w440, w438) -> (w446:T1)
                      n124 = Bundle By Name(cluster=w446, "FilePath"=w444, "Processed"=TRUE) -> (w445:T1)
                      n125 = in-place-array #1(w445) -> (w441:T1[])  [unwired: 1 out]
                    }
                  }
                  frame False {
                  }
                }
                n126 = case shown="True" w397 {
                  tunnel: w406 -> [w414 w427]
                  tunnel: [w414 w426] -> w407
                  tunnel: w404 -> [w413 w419]
                  tunnel: [w413 w425] -> w405
                  tunnel: w398 -> [_ w423]
                  tunnel: w392 -> [_ w420]
                  frame False {
                  }
                  frame True {
                    n127 = Search and Replace String(input string=w420, search string="clx", replace string="emg" ("replace string (\"\")"), error in=w419) -> (result string=w417:string, error out=w418:errorcluster)  [unwired: 4 in, 2 out]
                    n128 = local read "EMGmean"() -> (w422:dbl[][])
                    n129 = local read "Overwrite"() -> (w421:bool)
                    n130 = local read "EMGstd"() -> (w424:dbl[][])
                    n131 = call "WriteResFile.vi"("EMGstd"=w424, "EMGmean"=w422, "Overwrite"=w421, "error in (no error)"=w418, "New File Name"=w417, "Folder Path"=w423, "EMG in"=w427) -> ("error out"=w425:errorcluster, "EMG out"=w426:refnum<class "EMG.lvclass">)  [unwired: 3 in]
                  }
                }
              }
              event "Next": Value Change {
                # "OPEN NEXT FILE: Increament file list value"
                n132 = event-data() -> ()  [unwired: 1 in, 5 out]
                n133 = property on="File List" class="LstBox (strict)"(error in=w452) -> (error out=w453:errorcluster, "Value"=w458:i32)  [unwired: 1 in, 1 out]
                n134 = Array Size(array=w455) -> (size(s)=w456:i32)
                n135 = Increment(x=w458) -> (x+1=w454:i32)
                n136 = Less Or Equal?(x=w456, y=w454) -> (x <= y?=w460:bool)
                n137 = Select(t=0 ("f"), s=w460, f=w454) -> (s? t:f=w459:i32)
                n138 = property on="File List" class="LstBox (strict)"(error in=w453, "Val(Sgnl)"=w459) -> (error out=w451:errorcluster)  [unwired: 1 in, 1 out]
              }
              event "Graph-AnklePos": Scale Range Change; "Graph-EMG": Autoscale Range Change {
                # "Synchronize X Scale change of different plots"
                n139 = event-data() -> ("Source"=w465:T5, "CtlRef"=w467:refnum<vi>, "Kind"=w466:enum16{"X-Scale", "Y-Scale", "Z-Scale"}, "NewRange"=w468:T6)  [unwired: 1 in, 4 out]
                n140 = case shown="\"X-Scale\", Default" w466 {
                  tunnel: w468 -> [w475 _]
                  tunnel: w467 -> [w477 _]
                  tunnel: w465 -> [_ _]
                  frame "X-Scale", Default {
                    n141 = control-ref of="Graph-AnklePos"() -> ()  [unwired: 1 out]
                    n142 = property class="WFGraph (strict)"(reference=w477) -> ("Label.Text"=w476:string)  [unwired: 1 in, 2 out]
                    n143 = control-ref of="Graph-JointAngles"() -> ()  [unwired: 1 out]
                    n144 = control-ref of="Graph-EMG"() -> ()  [unwired: 1 out]
                    n145 = case shown="\"Graph-AnklePos\"" w476 {
                      tunnel: w475 -> [_ w483 w494]
                      frame Default {
                      }
                      frame "Graph-AnklePos" {
                        n146 = Unbundle By Name(w483) -> ("Minimum"=w482:dbl, "Maximum"=w481:dbl)
                        n147 = control-ref of="Graph-JointAngles"() -> (w485:refnum<vi>)
                        n148 = local read "Scale(x1)"() -> (w478:u16)
                        n149 = property class="WFGraph (strict)"(reference=w485, "XScale.Range"=w483) -> ()  [unwired: 1 in, 2 out]
                        n150 = control-ref of="Graph-EMG"() -> (w484:refnum<vi>)
                        n151 = Multiply(x=w478, y=w482) -> (x*y=w479:dbl)
                        n152 = Multiply(x=w478, y=w481) -> (x*y=w480:dbl)
                        n153 = property class="WFGraph (strict)"(reference=w484, "XScale.Minimum"=w479, "XScale.Maximum"=w480) -> ()  [unwired: 1 in, 2 out]
                      }
                      frame "Graph-EMG" {
                        n154 = Unbundle By Name(w494) -> ("Minimum"=w493:dbl, "Maximum"=w491:dbl)
                        n155 = local read "Scale(x1)"() -> (w492:u16)
                        n156 = control-ref of="Graph-AnklePos"() -> (w490:refnum<vi>)
                        n157 = Divide(x=w493, y=w492) -> (x/y=w487:dbl)
                        n158 = Divide(x=w491, y=w492) -> (x/y=w486:dbl)
                        n159 = property class="WFGraph (strict)"(reference=w490, "XScale.Minimum"=w487, "XScale.Maximum"=w486) -> (error out=w488:errorcluster)  [unwired: 1 in, 1 out]
                        n160 = control-ref of="Graph-JointAngles"() -> (w489:refnum<vi>)
                        n161 = property class="WFGraph (strict)"(reference=w489, error in=w488, "XScale.Minimum"=w487, "XScale.Maximum"=w486) -> ()  [unwired: 2 out]
                      }
                    }
                  }
                  frame "Y-Scale", "Z-Scale" {
                  }
                }
              }
              event "EMGmean-display": Plot Attribute Change {
                n162 = event-data() -> ()  [unwired: 1 in, 8 out]
                n163 = local read "MuscleNum"() -> (w503:i32)
                n164 = control-ref of="EMGmean-display"() -> (w507:refnum<vi>)
                n165 = control-ref of="Graph-EMG"() -> (w502:refnum<vi>)
                n166 = property class="EMG.lvclass"(reference=w501, error in=w499) -> (reference out=w500:refnum<class "EMG.lvclass">, error out=w498:errorcluster, "DataAccess:MuscleNumber"=w497:i32)
                n167 = for {
                  N: w503 -> [_]
                  tunnel: w507 -> [w516]
                  tunnel: w502 -> [w515]
                  tunnel: w497 -> [w508]
                  shift-right: [w514] -> w495
                  shift-left: w496 -> [w510]
                  i -> [w511]
                  n168 = property class="WFGraph (strict)"(reference=w516, error in=w510, "Active Plot"=w511) -> (error out=w517:errorcluster, "Plot.Visible?"=w513:bool, "Plot.Plot Name"=w509:string)  [unwired: 1 out]
                  n169 = Add(x=w511, y=w508) -> (x+y=w512:i32)
                  n170 = property class="WFGraph (strict)"(reference=w515, error in=w517, "Active Plot"=w511, "Plot.Visible?"=w513, "Plot.Plot Name"=w509, "Active Plot"=w512, "Plot.Visible?"=w513, "Plot.Plot Name"=w509) -> (error out=w514:errorcluster)  [unwired: 1 out]
                }
              }
              event "EMGmean-shift": Value Change {
                n171 = event-data() -> ()  [unwired: 1 in, 6 out]
              }
              event "EMG Y scale": Value Change {
                n172 = event-data() -> ()  [unwired: 1 in, 6 out]
                n173 = Negate(x="EMG Y scale") -> (-x=w525:i32)
                n174 = property on="Graph-EMG" class="WFGraph (strict)"("YScale.Minimum"=w525, "YScale.Maximum"="EMG Y scale") -> ()  [unwired: 2 in, 2 out]
              }
            }
          }
        }
        n175 = local read "CutVar"() -> (w38:enum16{"3D-x", "2D-x"})
        n176 = property class="EMG.lvclass"(reference=w55, error in=w53) -> (reference out=w54:refnum<class "EMG.lvclass">, error out=w52:errorcluster, "DataAccess:Time"=w14:dbl[], "DataAccess:MuscleDataFiltered"=w10:dbl[][])
        n177 = for {
          tunnel: w65 -> [w543] mode=indexing
          tunnel: [w537] -> w45 mode=indexing
          i -> [w536]
          n178 = Unbundle By Name(w543) -> ("Processed"=w535:bool, "FilePath"=w542:path, "EMGPath"=w541:path)
          n179 = Select(t=u32 9868950, s=w535, f=u32 16448250) -> (s? t:f=w532:u32)
          n180 = Strip Path(path=w542) -> (name=w540:string)  [unwired: 1 out]
          n181 = Strip Path(path=w541) -> (name=w539:string)  [unwired: 1 out]
          n182 = property on="File List" class="LstBox (strict)"("Active Row"=w536, "CellBG"=w532) -> ()  [unwired: 2 in, 2 out]
          n183 = Concatenate Strings(w540, "\n-> " ("string"), w539) -> (w537:string)
        }
        n184 = call "GetCutData.vi"("error in (no error)"=w42, "CutVar"=w38, "CAlexData"=w40) -> ("error out"=w41:errorcluster, "Time"=w15:dbl[], "CAlexData out"=w43:refnum<class "CAlex2_Data.lvclass">, "MarkingVar3"=w36:dbl[][])  [unwired: 4 in, 1 out]
        n185 = call "Mark_GetBEMark.vi"("error in (no error)"=w41, "ExpData In"=w43) -> ("error out"=w59:errorcluster, "End"=w16:dbl[], "Begin"=w17:dbl[], "ExpData Out"=w44:refnum<class "CAlex2_Data.lvclass">)  [unwired: 5 in, 1 out]
        n186 = Array Size(array=w16) -> (size(s)=w49:i32)
        n187 = Array Size(array=w17) -> (size(s)=w50:i32)
        n188 = control-ref of="Graph-AnklePos"() -> (w19:refnum<vi>)
        n189 = call "Cut&Average.vi"("Data"=w36, "Time"=w15, "End"=w16, "Begin"=w17) -> ("Dilated"=w58:dbl[][][], "Mean"=w37:dbl[][], "CuttedData-Concatenated"=w35:dbl[][])  [unwired: 2 in, 3 out]
        n190 = call "Cut&Average.vi"("Data"=w10, "Time"=w14, "End"=w16, "Begin"=w17) -> ("Std"=→"EMGstd":dbl[][], "Mean"=w13:dbl[][])  [unwired: 2 in, 4 out]
        "EMGmean" <- w13
        n191 = Add(x=w49, y=w50) -> (x+y=w48:i32)
        n192 = call "AddGraphAnnotation.vi"("Input Type (Time)"=w18, "WaveformGraph in"=w19, "Time"=w15, "Valleys  (Yellow)"=w16, "Peaks (Red)"=w17) -> ("error out"=w21:errorcluster)  [unwired: 5 in, 1 out]
        n193 = Divide(x=w48, y=2) -> (x/y=→"Cycle#":dbl)
        n194 = Index Array(array=w58, index (dim 1)=0 ("disabled index (row)")) -> (element=→"AnglesCutted":dbl[][])  [unwired: 2 in]
        n195 = for {
          tunnel: w13 -> [w69] mode=indexing
          tunnel: "EMGmean-shift" -> [w70]
          tunnel: [w68] -> w11 mode=indexing
          n196 = Rotate 1D Array(1:w69, 2:w70) -> (0:w68:dbl[])
        }
        "EMGmean-display" <- w11
        n197 = control-ref of="Graph-JointAngles"() -> (w20:refnum<vi>)
        n198 = property on="File List" class="LstBox (strict)"("Item Names"=w45) -> ()  [unwired: 2 in, 2 out]
        n199 = call "AddGraphAnnotation.vi"("error in (no error)"=w21, "Input Type (Time)"=w18, "WaveformGraph in"=w20, "Time"=w15, "Valleys  (Yellow)"=w16, "Peaks (Red)"=w17) -> ("error out"=w22:errorcluster)  [unwired: 4 in, 1 out]
        n200 = control-ref of="Graph-EMG"() -> (w23:refnum<vi>)
        n201 = call "AddGraphAnnotation.vi"("error in (no error)"=w22, "Input Type (Time)"=w18, "WaveformGraph in"=w23, "Time"=w14, "Valleys  (Yellow)"=w16, "Peaks (Red)"=w17) -> ()  [unwired: 4 in, 2 out]
        n202 = Index Array(array=w35, index (row) #1=0 ("index (row)"), index (row) #2=1 ("index (row)")) -> (element #1=w28:dbl[], element #2=w27:dbl[])  [unwired: 2 in]
        n203 = Index Array(array=w37, index (row) #1=0 ("index (row)"), index (row) #2=1 ("index (row)")) -> (element #1=w33:dbl[], element #2=w34:dbl[])  [unwired: 2 in]
        n204 = Bundle("CuttedData-Concatenated"=w28, "CuttedData-Concatenated"=w27) -> (w24:T7)  [unwired: 1 in]
        n205 = Bundle("Mean"=w33, "Mean"=w34) -> (w25:cluster{"Mean":dbl[], "Mean":dbl[]})  [unwired: 1 in]
        n206 = Build Array(w25, w24) -> (→"GaitTraj":T8)
      }
    }
  }
